vi "kkk.vi"() -> ()   [LabVIEW 2015]
uses:
  <vilib>/eio/EIONode/EIONode.xnode
  <vilib>/rvi/eio/common/nirviEmuTemplateMethod_errors.vi
panel:
  in  "led4":bool
  in  "led1":bool
  in  "led3":bool
  in  "led2":bool
  out "Boolean 4":bool
  out "Boolean 3":bool
  out "Boolean 2":bool
  out "Boolean":bool
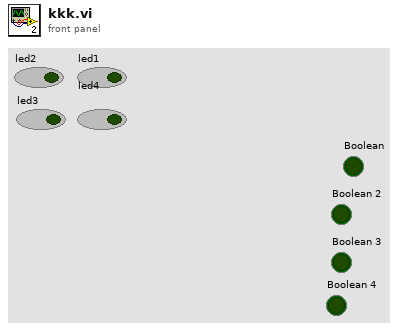
[diagram p1: front panel]
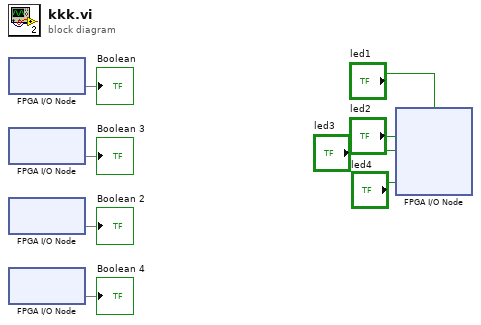
[diagram p0: block diagram]
diagram:
  n1 = xnode "FPGA I/O Node"() -> ("DIO16"=→"Boolean")  [unwired: 1 in, 1 out]
  n2 = xnode "FPGA I/O Node"() -> ("DIO15"=→"Boolean 3")  [unwired: 1 in, 1 out]
  n3 = xnode "FPGA I/O Node"() -> ("DIO14"=→"Boolean 2")  [unwired: 1 in, 1 out]
  n4 = xnode "FPGA I/O Node"() -> ("DIO13"=→"Boolean 4")  [unwired: 1 in, 1 out]
  n5 = xnode "FPGA I/O Node"("DIO4"="led2", "DIO5"="led3", "DIO6"="led1", "DIO7"="led4") -> ()  [unwired: 4 in, 4 out]
